vi "_FPGA Check Vacuum.vi"() -> (2 "Vac OK":bool, 3 "Source OK":bool, 4 "Stop":bool, 5 "Shutdown":bool)   [LabVIEW 2015]
uses:
  _RT Global.vi
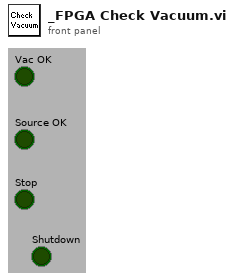
[diagram p1: front panel]
types:
  T1 = typedef "_RT Startup Options.ctl" = cluster{"Door":bool, "Curtain":bool, "Pressure":bool, "Turbo":bool, "SysPoll":bool, "GasFlag":bool}
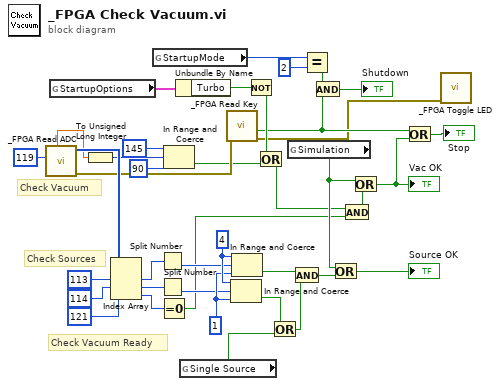
[diagram p0: block diagram]
diagram:
  w26 = u16 4 ("upper limit")
  w25 = u16 1 ("lower limit")
  # "Check Vacuum Ready"
  # "Check Sources"
  # "Check Vacuum"
  n1 = call "_FPGA Read ADC.vi"("ADC Channel (64)"=119) -> ("error out"=w27:errorcluster, "ADC Values"=w33:i32[], "Raw Reading"=w7:sgl)  [unwired: 2 in, 4 out]
  n2 = global read "_RT Global.vi" "StartupOptions"() -> (w38:T1)
  n3 = To Unsigned Long Integer(number=w7) -> (unsigned 32bit integer=w8:u32)
  n4 = Index Array(array=w33, index #1=113 ("ADC Channel (64)"), index #2=114 ("ADC Channel (64)"), index #3=121 ("ADC Channel (64)")) -> (element #1=w35:i32, element #2=w34:i32, element #3=w29:i32)
  n5 = global read "_RT Global.vi" "StartupMode"() -> (w6:u8)
  n6 = Split Number(x=w35) -> (lo(x)=w24:u16)  [unwired: 1 out]
  n7 = Split Number(x=w34) -> (lo(x)=w23:u16)  [unwired: 1 out]
  n8 = Equal To 0?(x=w29) -> (x = 0?=w9:bool)
  n9 = In Range and Coerce(upper limit=u32 145, x=w8, lower limit=u32 90) -> (In Range?=w12:bool)  [unwired: 1 out]
  n10 = Unbundle By Name(w38) -> ("Turbo"=w39:bool)
  n11 = global read "_RT Global.vi" "Single Source"() -> (w18:bool)
  n12 = call "_FPGA Read Key.vi"("error in (no error)"=w27) -> ("error out"=w1:errorcluster, "Key Pressed"=w3:bool)  [unwired: 4 in, 2 out]
  n13 = In Range and Coerce(upper limit=w26, x=w23, lower limit=w25) -> (In Range?=w17:bool)  [unwired: 1 out]
  n14 = In Range and Coerce(upper limit=w26, x=w24, lower limit=w25) -> (In Range?=w19:bool)  [unwired: 1 out]
  n15 = Not(x=w39) -> (.not. x?=w11:bool)
  n16 = Or(x=w11, y=w12) -> (x .or. y?=w10:bool)
  n17 = Or(x=w17, y=w18) -> (x .or. y?=w16:bool)
  n18 = global read "_RT Global.vi" "Simulation"() -> (w14:bool)
  n19 = And(x=w19, y=w16) -> (x .and. y?=w20:bool)
  n20 = Equal?(x=w6, y=u8 2) -> (x = y?=w4:bool)
  n21 = And(x=w4, y=w3) -> (x .and. y?=→"Shutdown":bool)
  n22 = Or(x=w14, y=w20) -> (x .or. y?=→"Source OK":bool)
  n23 = And(x=w10, y=w9) -> (x .and. y?=w13:bool)
  n24 = Or(x=w14, y=w13) -> (x .or. y?=w21:bool)
  "Vac OK" <- w21
  n25 = Or(x=w3, y=w21) -> (x .or. y?=→"Stop":bool)
  n26 = call "_FPGA Toggle LED.vi"("error in (no error)"=w1) -> ()  [unwired: 4 in, 4 out]
